vi "Control Type.vi"(11 "Valve in":refnum<class "PeriodicControl.lvclass">) -> (2 "Valve Type":string)   [LabVIEW 2020, in "VolatusControl.lvlib" / "PeriodicControl.lvclass"]
uses:
  PeriodicControl.lvclass
  PeriodicControl.lvclass/PeriodicControl.ctl
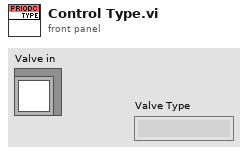
[diagram p1: front panel]
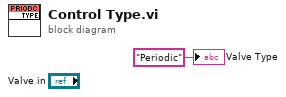
[diagram p0: block diagram]
diagram:
  "Valve Type" <- "Periodic" ("Valve Type")
